vi "Initialise.vi"(8 "error in (no error)":errorcluster) -> (0 "error out":errorcluster)   [LabVIEW 2015, in "Resource Manager.lvclass"]
uses:
  Resource Manager.lvclass
  Globals.vi
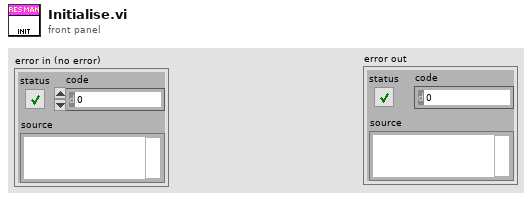
[diagram p1: front panel]
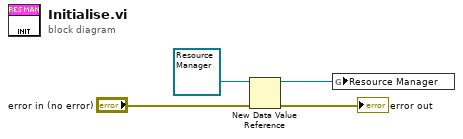
[diagram p0: block diagram]
diagram:
  n1 = New Data Value Reference(data value=refnum<class "Resource Manager.lvclass"> refnum ("Texture Manager in"), error in="error in (no error)") -> (data value reference=w4:refnum<data-value>, error out=→"error out":errorcluster)
  n2 = global write "Globals.vi" "Resource Manager"(w4) -> ()
